vi "Handle Debug Data.vi"(7 "Action":enum16{"Send", "Receive", "Request", "Response"}(ring), 8 "error in (no error)":errorcluster, 9 "Message Data":variant, 10 "Message":string, 11 "Process In":refnum<class "Process.lvclass">) -> (0 "error out":errorcluster, 3 "Process Out":refnum<class "Process.lvclass">)   [LabVIEW 2020, in "Process.lvclass"]
doc: "Record data for debugging purposes."
uses:
  Process.lvclass
  Process.lvclass/Process.ctl
  Logging/Logging.lvclass
  C:/git/astemes-triarc-framework/source/Framework/Base/Base.lvclass
  C:/git/astemes-triarc-framework/source/Framework/Process/Process.lvclass
  C:/git/astemes-triarc-framework/source/Framework/Error Handler Interface/Error Handler Interface.lvclass
  C:/git/astemes-triarc-framework/source/Framework/Logging/Logging.lvclass
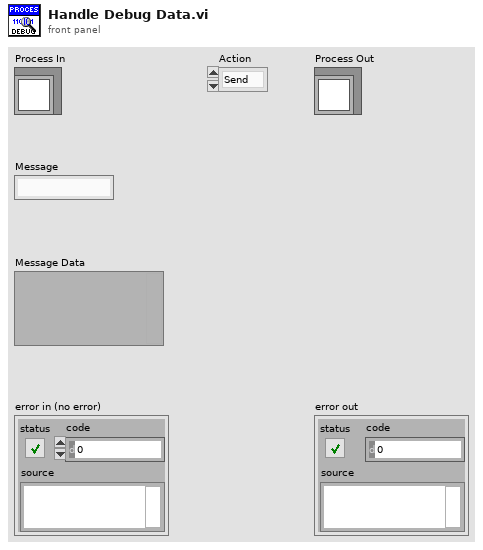
[diagram p1: front panel]
types:
  T1 = cluster{"Action":string, "Call Chain":string, "Process":string, "Message":string, "Message Data":variant, "Time":dbl}
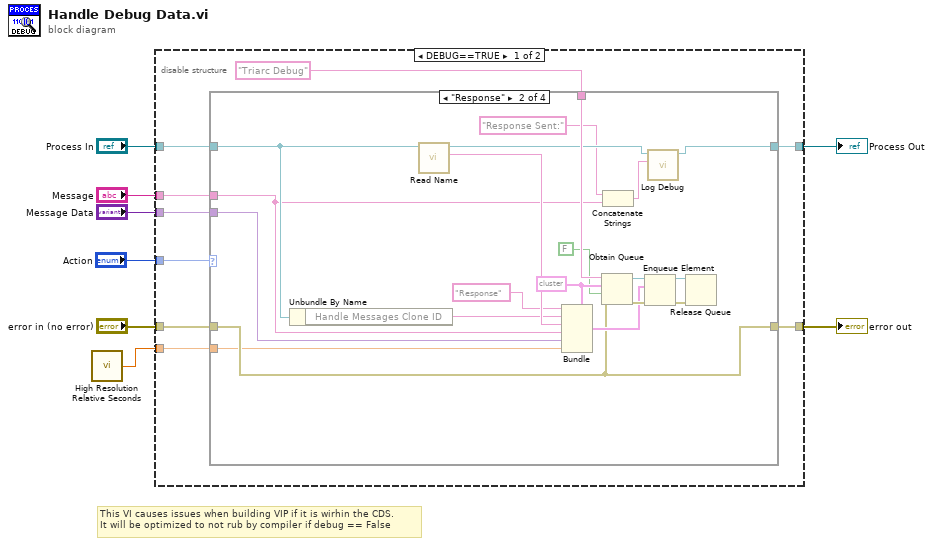
[diagram p0: block diagram]
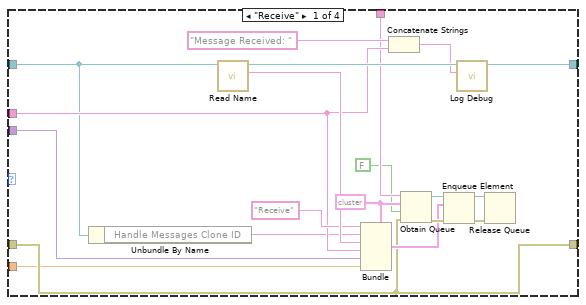
[diagram p2: hidden frame]
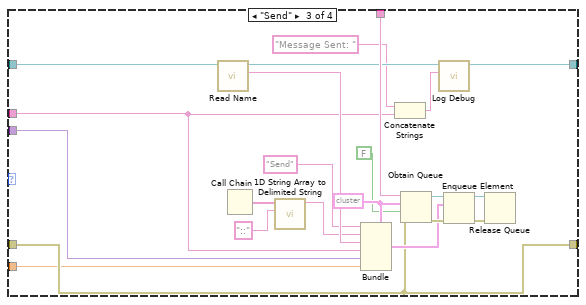
[diagram p3: hidden frame]
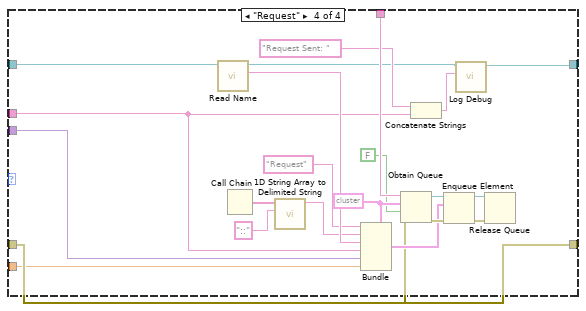
[diagram p4: hidden frame]
diagram:
  # "This VI causes issues when building VIP if it is wirhin the CDS.\nIt will be optimized to not rub by compiler if debug == False"
  n1 = call <vilib>:"High Resolution Relative Seconds.vi"() -> ("relative seconds"=w1:dbl)
  n2 = disable-structure shown="DEBUG==TRUE" {
    disable-tunnel: "Message" -> [w15 _]
    disable-tunnel: "Message Data" -> [w17 _]
    disable-tunnel: [w16 w103] -> w5
    disable-tunnel: "Process In" -> [w14 w103]
    disable-tunnel: [w13 w102] -> w6
    disable-tunnel: "error in (no error)" -> [w12 w102]
    disable-tunnel: "Action" -> [w11 _]
    disable-tunnel: w1 -> [w9 _]
    frame condition #0 {
      n3 = case shown="\"Response\"" w11 {
        tunnel: w17 -> [w29 w49 w69 w91]
        tunnel: [w27 w40 w61 w81] -> w16
        tunnel: w15 -> [w24 w38 w59 w80]
        tunnel: w14 -> [w23 w48 w68 w90]
        tunnel: [w19 w44 w64 w87] -> w13
        tunnel: w12 -> [w19 w44 w64 w87]
        tunnel: "Triarc Debug" ("name (unnamed)") -> [w21 w46 w66 w88]
        tunnel: w9 -> [w18 w43 w63 w85]
        frame "Receive" {
          w36 = T1 {"Action"="", "Call Chain"="", "Process"="", "Message"="", "Message Data"=variant, "Time"=0.0} ("output cluster")
          n4 = Unbundle By Name(w23) -> ("Handle Messages Clone ID"=w22:string)
          n5 = call "Read Name.vi"("Process In"=w23) -> ("Qualified Name"=w37:string, "Process Out"=w28:refnum<class "Process.lvclass">)  [unwired: 7 in, 2 out]
          n6 = Bundle(cluster=w36, "Action"="Receive", "Call Chain"=w22, "Process"=w37, "Message"=w24, "Message Data"=w29, "Time"=w18) -> (w33:T1)
          n7 = Concatenate Strings("Message Received: " ("name (unnamed)"), w24) -> (w25:string)
          n8 = Obtain Queue(name (unnamed)=w21, element data type=w36, create if not found? (T)=FALSE, error in (no error)=w19) -> (queue out=w35:refnum<queue>, error out=w34:errorcluster)  [unwired: 1 in, 1 out]
          n9 = Enqueue Element(queue=w35, element=w33, error in (no error)=w34) -> (queue out=w32:refnum<queue>, error out=w31:errorcluster)  [unwired: 1 in, 1 out]
          n10 = call "Log Debug.vi"("Message"=w25, "Logging In"=w28) -> ("Logging Out"=w27:refnum<class "Process.lvclass">)  [unwired: 8 in, 1 out]
          n11 = Release Queue(queue=w32, error in (no error)=w31) -> ()  [unwired: 1 in, 3 out]
        }
        frame "Response" {
          w56 = T1 {"Action"="", "Call Chain"="", "Process"="", "Message"="", "Message Data"=variant, "Time"=0.0} ("output cluster")
          n12 = Unbundle By Name(w48) -> ("Handle Messages Clone ID"=w47:string)
          n13 = call "Read Name.vi"("Process In"=w48) -> ("Qualified Name"=w57:string, "Process Out"=w41:refnum<class "Process.lvclass">)  [unwired: 7 in, 2 out]
          n14 = Bundle(cluster=w56, "Action"="Response", "Call Chain"=w47, "Process"=w57, "Message"=w38, "Message Data"=w49, "Time"=w43) -> (w53:T1)
          n15 = Obtain Queue(name (unnamed)=w46, element data type=w56, create if not found? (T)=FALSE, error in (no error)=w44) -> (queue out=w55:refnum<queue>, error out=w54:errorcluster)  [unwired: 1 in, 1 out]
          n16 = Concatenate Strings("Response Sent:", w38) -> (w42:string)
          n17 = Enqueue Element(queue=w55, element=w53, error in (no error)=w54) -> (queue out=w52:refnum<queue>, error out=w51:errorcluster)  [unwired: 1 in, 1 out]
          n18 = call "Log Debug.vi"("Message"=w42, "Logging In"=w41) -> ("Logging Out"=w40:refnum<class "Process.lvclass">)  [unwired: 8 in, 1 out]
          n19 = Release Queue(queue=w52, error in (no error)=w51) -> ()  [unwired: 1 in, 3 out]
        }
        frame "Send" {
          w67 = T1 {"Action"="", "Call Chain"="", "Process"="", "Message"="", "Message Data"=variant, "Time"=0.0} ("output cluster")
          n20 = call "Read Name.vi"("Process In"=w68) -> ("Qualified Name"=w79:string, "Process Out"=w62:refnum<class "Process.lvclass">)  [unwired: 7 in, 2 out]
          n21 = Call Chain() -> (call chain=w78:string[])
          n22 = call <vilib>:"1D String Array to Delimited String.vi"("delimiter"="::", "string array"=w78) -> ("delimited string"=w76:string)  [unwired: 9 in]
          n23 = Bundle(cluster=w67, "Action"="Send", "Call Chain"=w76, "Process"=w79, "Message"=w59, "Message Data"=w69, "Time"=w63) -> (w73:T1)
          n24 = Concatenate Strings("Message Sent: " ("name (unnamed)"), w59) -> (w58:string)
          n25 = Obtain Queue(name (unnamed)=w66, element data type=w67, create if not found? (T)=FALSE, error in (no error)=w64) -> (queue out=w75:refnum<queue>, error out=w74:errorcluster)  [unwired: 1 in, 1 out]
          n26 = call "Log Debug.vi"("Message"=w58, "Logging In"=w62) -> ("Logging Out"=w61:refnum<class "Process.lvclass">)  [unwired: 8 in, 1 out]
          n27 = Enqueue Element(queue=w75, element=w73, error in (no error)=w74) -> (queue out=w72:refnum<queue>, error out=w71:errorcluster)  [unwired: 1 in, 1 out]
          n28 = Release Queue(queue=w72, error in (no error)=w71) -> ()  [unwired: 1 in, 3 out]
        }
        frame "Request" {
          w89 = T1 {"Action"="", "Call Chain"="", "Process"="", "Message"="", "Message Data"=variant, "Time"=0.0} ("output cluster")
          n29 = call "Read Name.vi"("Process In"=w90) -> ("Qualified Name"=w101:string, "Process Out"=w82:refnum<class "Process.lvclass">)  [unwired: 7 in, 2 out]
          n30 = Call Chain() -> (call chain=w100:string[])
          n31 = call <vilib>:"1D String Array to Delimited String.vi"("delimiter"="::", "string array"=w100) -> ("delimited string"=w98:string)  [unwired: 9 in]
          n32 = Bundle(cluster=w89, "Action"="Request", "Call Chain"=w98, "Process"=w101, "Message"=w80, "Message Data"=w91, "Time"=w85) -> (w95:T1)
          n33 = Obtain Queue(name (unnamed)=w88, element data type=w89, create if not found? (T)=FALSE, error in (no error)=w87) -> (queue out=w97:refnum<queue>, error out=w96:errorcluster)  [unwired: 1 in, 1 out]
          n34 = Concatenate Strings("Request Sent: " ("name (unnamed)"), w80) -> (w84:string)
          n35 = Enqueue Element(queue=w97, element=w95, error in (no error)=w96) -> (queue out=w94:refnum<queue>, error out=w93:errorcluster)  [unwired: 1 in, 1 out]
          n36 = call "Log Debug.vi"("Message"=w84, "Logging In"=w82) -> ("Logging Out"=w81:refnum<class "Process.lvclass">)  [unwired: 8 in, 1 out]
          n37 = Release Queue(queue=w94, error in (no error)=w93) -> ()  [unwired: 1 in, 3 out]
        }
      }
    }
    frame condition #1 (active) {
    }
  }
  "error out" <- w6
  "Process Out" <- w5
